vi "PlaySoundBelow50m.vi"   [LabVIEW 2014]
doc: "This VI demonstrates an asynchronous call and forget. When this VI is run, it asynchronously calls a target VI and will not wait for the results. This VI will run to completion while the target VI continues to run.\n\nThis example uses the Start Asynchronous Call method and the Open VI Reference option 0x80.\n\nWhen running this example, notice this VI finishes execution while the target VI continues to run."
uses:
  isPlaying.vi
panel:
  # "This Vi calls a warning using another thread to advoid delays using CheckOutBeep.wav"
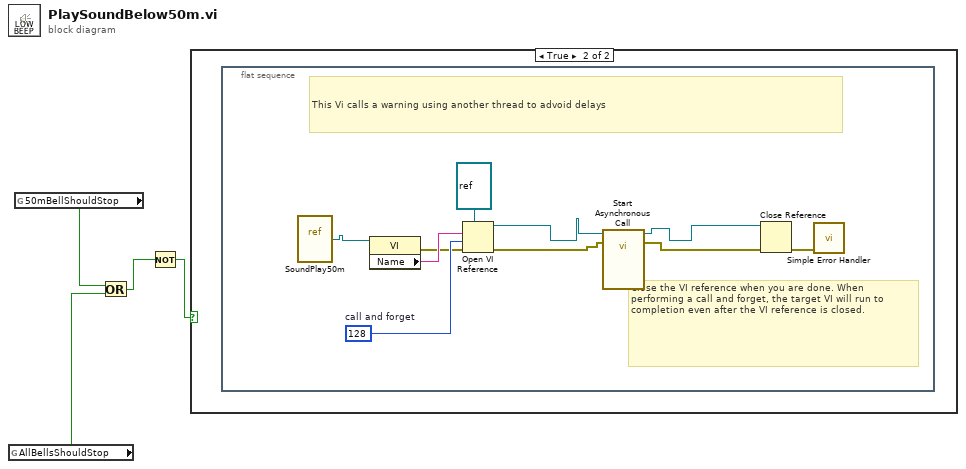
[diagram p0: block diagram]
diagram:
  n1 = global read "isPlaying.vi" "AllBellsShouldStop"() -> (w3:bool)
  n2 = global read "isPlaying.vi" "50mBellShouldStop"() -> (w4:bool)
  n3 = Or(x=w4, y=w3) -> (x .or. y?=w2:bool)
  n4 = Not(x=w2) -> (.not. x?=w1:bool)
  n5 = case shown="True" w1 {
    frame False {
    }
    frame True {
      n6 = flat-sequence {
        frame #0 {
          w14 = 128  # call and forget
          # "Close the VI reference when you are done. When performing a call and forget, the target VI will run to completion even after the VI reference is closed."
          # "This Vi calls a warning using another thread to advoid delays"
          n7 = vi-ref "SoundPlay50m.vi"() -> (w9:refnum<vi>)
          n8 = property class="VI"(reference=w9) -> (error out=w11:errorcluster, "Name"=w12:string)  [unwired: 1 in, 1 out]
          n9 = Open VI Reference(type specifier VI Refnum (for type only)=refnum<vi> refnum, vi path=w12, options=w14, error in (no error)=w11) -> (vi reference=w8:refnum<vi>, error out=w7:errorcluster)  [unwired: 2 in]
          n10 = call-by-ref "Start Asynchronous Call"(reference=w8, error in=w7) -> (reference out=w5:refnum<vi>, error out=w6:errorcluster)  [unwired: 1 in]
          n11 = Close Reference(reference=w5, error in (no error)=w6) -> (error out=w13:errorcluster)
          n12 = call <vilib>:"Simple Error Handler.vi"("error in (no error)"=w13) -> ()  [unwired: 4 in, 5 out]
        }
      }
    }
  }
